vi "Clean CCD.vi"(8 "error in (no error)":errorcluster, 11 "CCDCamera in":refnum<class "Simulated_CCD_Camera.lvclass">) -> (0 "error out":errorcluster, 3 "CCDCamera out":refnum<class "Simulated_CCD_Camera.lvclass">)   [LabVIEW 2018, in "Simulated_CCD_Camera.lvclass"]
uses:
  Simulated_CCD_Camera.lvclass
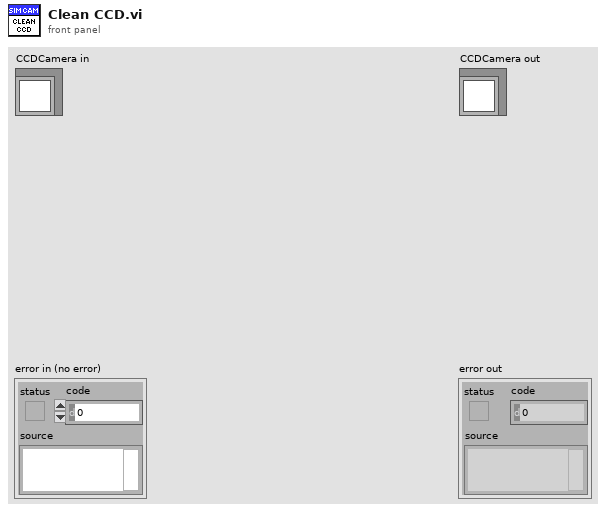
[diagram p1: front panel]
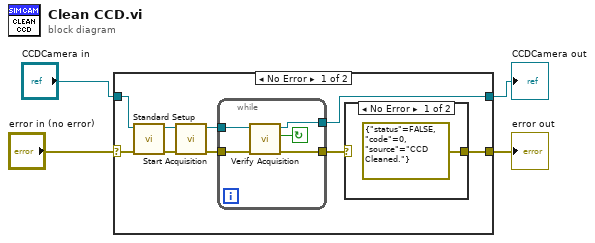
[diagram p0: block diagram]
diagram:
  n1 = case shown="No Error" "error in (no error)" {
    selector: "error in (no error)" -> [w9 w22]
    tunnel: "CCDCamera in" -> [w6 w21]
    tunnel: [w5 w21] -> w1
    tunnel: [w13 w22] -> w2
    frame No Error {
      n2 = call-dynamic "Standard Setup.vi"("error in (no error)"=w9, "CCDCamera in"=w6) -> ("error out"=w11:errorcluster, "CCDCamera out"=w10:refnum<class "Simulated_CCD_Camera.lvclass">)  [unwired: 8 in]
      n3 = call-dynamic "Start Acquisition.vi"("error in (no error)"=w11, "CCDCamera in"=w10) -> ("error out"=w8:errorcluster, "CCDCamera out"=w7:refnum<class "Simulated_CCD_Camera.lvclass">)  [unwired: 8 in]
      n4 = while {
        tunnel: [w19] -> w12
        tunnel: [w20] -> w5
        tunnel: w8 -> [w17]
        tunnel: w7 -> [w16]
        stop <- w18 continue-if-true
        n5 = call-dynamic "Verify Acquisition.vi"("error in (no error)"=w17, "CCDCamera in"=w16) -> ("error out"=w19:errorcluster, "Acquiring"=w18:bool, "CCDCamera out"=w20:refnum<class "Simulated_CCD_Camera.lvclass">)  [unwired: 7 in]
      }
      n6 = case shown="No Error" w12 {
        selector: w12 -> [_ w15]
        tunnel: [errorcluster {"status"=FALSE, "code"=0, "source"="CCD Cleaned."} ("error IO") w15] -> w13
        frame No Error {
        }
        frame Error {
        }
      }
    }
    frame Error {
    }
  }
  "error out" <- w2
  "CCDCamera out" <- w1
